vi "Exposure time.vi"(4 "MASTER in":T1 {"Image data"."Color Palette" items=["Grayscale U8", "False Color", "Overexposed"]; "Image data"."Exposure time [us]" format="%#_10g"; "Queue"."Initial time [s]" format="%_19f"; "Queue"."Raw data [V]\n(all samples)" format="%0.2f"; "Queue"."Timestamp [s]" format="%_19f"}) -> (1 "MASTER out":T1 {"Image data"."Color Palette" items=["Grayscale U8", "False Color", "Overexposed"]; "Image data"."Exposure time [us]" format="%#_10g"; "Queue"."Initial time [s]" format="%_19f"; "Queue"."Raw data [V]\n(all samples)" format="%0.2f"; "Queue"."Timestamp [s]" format="%_19f"})   [LabVIEW 2020]
uses:
  MASTER.ctl
  Constants.ctl
  QBundle.ctl
  Queue.ctl
  Image data.ctl
  <vilib>/userdefined/High Color/IMAQdx.ctl
  <vilib>/vision/Image Controls.llb/IMAQ Image.ctl
  Image QBundle.ctl
  <resource>/objmgr/imaqdx.rc
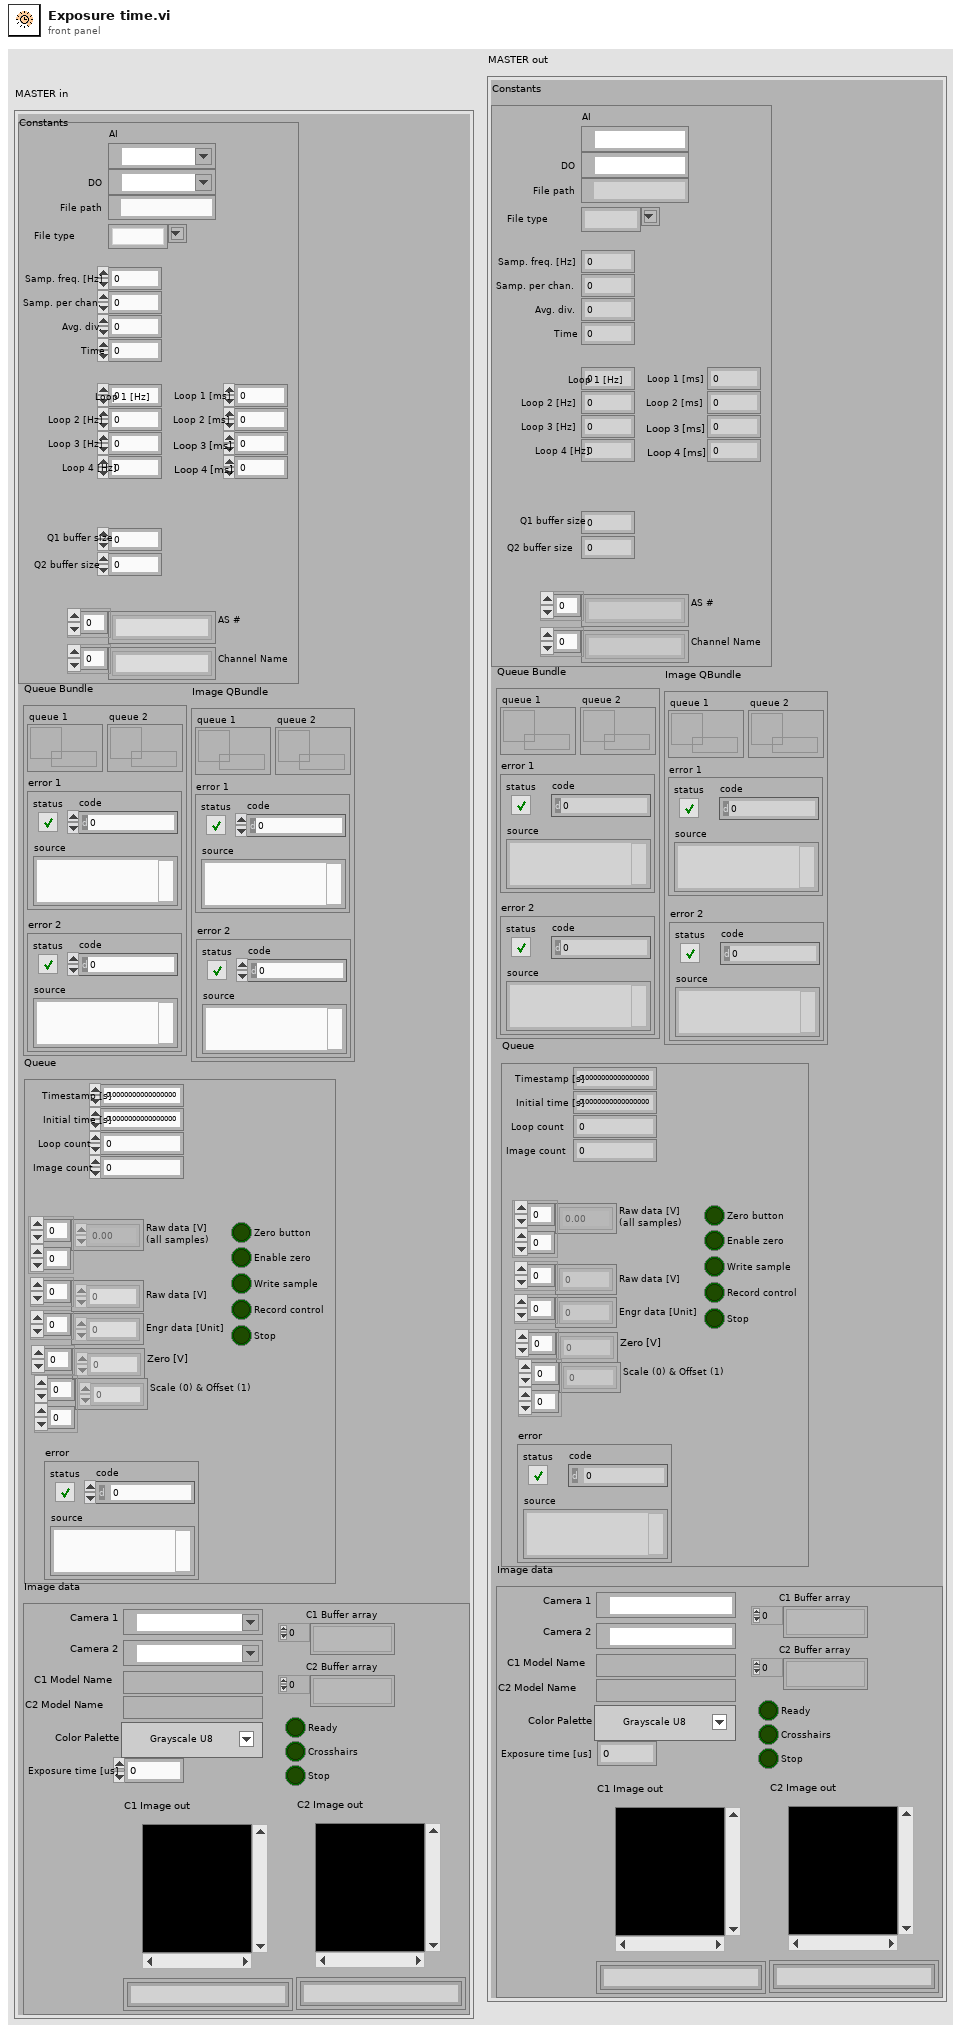
[diagram p1: front panel]
types:
  T1 = typedef "MASTER.ctl" = cluster{"Constants":T2, "Queue Bundle":T3, "Queue":T4, "Image data":T5, "Image QBundle ":T8}
  T2 = typedef "Constants.ctl" = cluster{"Time":u16, "Samp. freq. [Hz]":dbl, "Samp. per chan.":i32, "Avg. div.":i32, "File path":path, "AI":refnum<k21>, "Loop 1 [Hz]":dbl, "Loop 2 [Hz]":dbl, "Loop 3 [Hz]":dbl, "Loop 1 [ms]":dbl, "Loop 2 [ms]":dbl, "Loop 3 [ms]":dbl, "Q1 buffer size":i32, "Q2 buffer size":i32, "File type":string, "Loop 4 [Hz]":dbl, "Loop 4 [ms]":dbl, "Channel Name":string[], "AS #":string[], "DO":refnum<k21>}
  T3 = typedef "QBundle.ctl" = cluster{"queue 1":refnum<queue>, "error 1":errorcluster, "queue 2":refnum<queue>, "error 2":errorcluster}
  T4 = typedef "Queue.ctl" = cluster{"Enable zero":bool, "Engr data [Unit]":dbl[], "Zero button":bool, "Zero [V]":dbl[], "Timestamp [s]":dbl, "Write sample":bool, "Record control":bool, "Stop":bool, "error":errorcluster, "Raw data [V]\n(all samples)":dbl[][], "Raw data [V]":dbl[], "Loop count":i64, "Initial time [s]":dbl, "Scale (0) & Offset (1)":dbl[][], "Image count":dbl}
  T5 = typedef "Image data.ctl" = cluster{"Camera 1":T6, "Camera 2":T6, "C1 Image out ":T7, "C2 Image out":T7, "C1 Model Name":string, "C2 Model Name":string, "Exposure time [us]":dbl, "Color Palette":u16, "C1 Buffer array":T7[], "Ready":bool, "C2 Buffer array":T7[], "Crosshairs":bool, "Stop":bool}
  T6 = typedef "IMAQdx.ctl" = refnum<k21>
  T7 = typedef "IMAQ Image.ctl" = refnum<image>
  T8 = typedef "Image QBundle.ctl" = cluster{"queue 1":refnum<queue>, "error 1":errorcluster, "queue 2":refnum<queue>, "error 2":errorcluster}
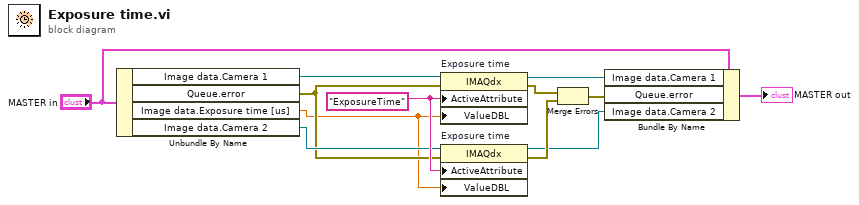
[diagram p0: block diagram]
diagram:
  w8 = "ExposureTime" ("ActiveAttribute")
  n1 = Unbundle By Name("MASTER in") -> ("Image data.Camera 1"=w12:T6, "Queue.error"=w6:errorcluster, "Image data.Exposure time [us]"=w5:dbl, "Image data.Camera 2"=w7:T6)
  n2 = property on="Exposure time" class="IMAQdx"(reference=w12, error in=w6, "ActiveAttribute"=w8, "ValueDBL"=w5) -> (reference out=w9:T6, error out=w4:errorcluster)
  n3 = property on="Exposure time" class="IMAQdx"(reference=w7, error in=w6, "ActiveAttribute"=w8, "ValueDBL"=w5) -> (reference out=w1:T6, error out=w2:errorcluster)
  n4 = Merge Errors(w4, w2) -> (w3:errorcluster)
  n5 = Bundle By Name(cluster="MASTER in", "Image data.Camera 1"=w9, "Queue.error"=w3, "Image data.Camera 2"=w1) -> (→"MASTER out":T1)
